vi "Set target speed.vi"(6 "Speed":i32(knob) scale=-200.0..200.0, 7 "timeout (1s)":dbl=1.0 min=0.0, 8 "error in (no error)":errorcluster, 11 "SDO object in":refnum<k20>) -> (0 "error out":errorcluster, 1 "completion code":u32, 3 "SDO object out":refnum<k20>)   [LabVIEW 2016]
uses:
  <vilib>/CANopenLib/CANOPEN.llb/CANopen SDO Write [I32].vi
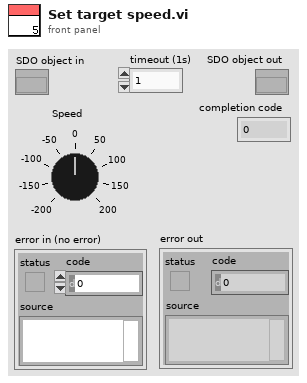
[diagram p1: front panel]
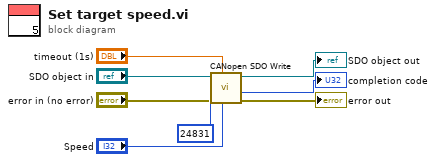
[diagram p0: block diagram]
diagram:
  n1 = call-poly <vilib>:"CANopen SDO Write.vi"("I32 data"="Speed", "timeout (1s)"="timeout (1s)", "error in (no error)"="error in (no error)", "object index"=u16 24831, "SDO object in"="SDO object in") -> ("error out"=→"error out":errorcluster, "completion code"=→"completion code":u32, "SDO object out"=→"SDO object out":refnum<k20>)  [unwired: 4 in]
